vi "intensity_function_derivatives.vi"(6 "theta_min":dbl, 8 "theta":dbl, 9 "C":dbl, 10 "B":dbl, 11 "A":dbl) -> (0 "dThetaMin":dbl, 1 "dC":dbl, 2 "dB":dbl, 3 "dA":dbl)   [LabVIEW 2019]
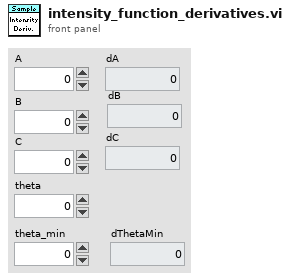
[diagram p1: front panel]
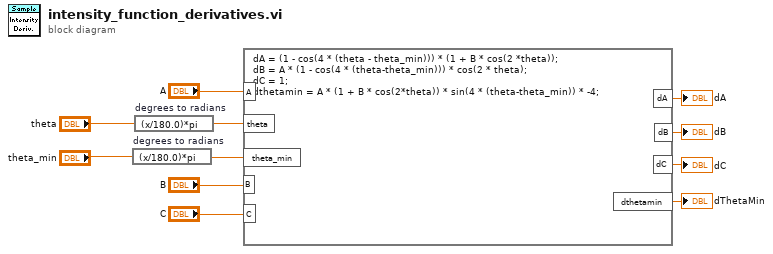
[diagram p0: block diagram]
diagram:
  n1 = expression code="(x/180.0)*pi" "degrees to radians"("theta_min") -> (w6:dbl)
  n2 = expression code="(x/180.0)*pi" "degrees to radians"("theta") -> (w7:dbl)
  n3 = formula code="dA = (1 - cos(4 * (theta - theta_min))) * (1 + B * cos(2 *theta));\ndB = A * (1 - cos(4 * (theta-theta_min))) * cos(2 * theta);\ndC = 1;\ndthetamin = A * (1 + B * cos(2*theta)) * sin(4 * (theta-theta_min)) * -4;"("A"="A", "theta"=w7, "theta_min"=w6, "B"="B", "C"="C") -> ("dA"=→"dA":dbl, "dB"=→"dB":dbl, "dC"=→"dC":dbl, "dthetamin"=→"dThetaMin":dbl)
